vi "Global Chart List.vi"(7 "Action":T1=enum."Append to Charts", 10 "Value":dbl, 11 "Chart Ref":refnum<class "LQChart.lvclass">) -> ()   [LabVIEW 2014]
doc: "An Action Engine that registers and updates the global list of charts, which are created dynamically (at run-time) in this application.\n\n\nCopyright (c) 2019 Sze Howe Koh.\nThis code is licensed under the MIT license."
uses:
  Global Chart List Action.ctl
  <vilib>/addons/LQ/LQ Extras/LQChart/LQChart.lvclass
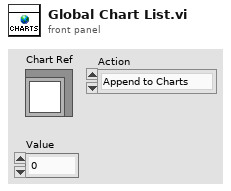
[diagram p1: front panel]
types:
  T1 = typedef "Global Chart List Action.ctl" = enum16{"Clear", "Register Chart", "Append to Charts"}
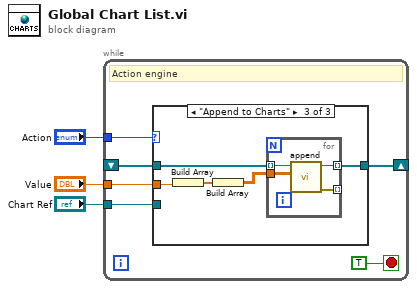
[diagram p0: block diagram]
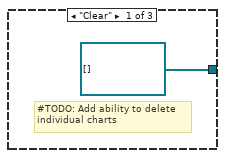
[diagram p2: hidden frame]
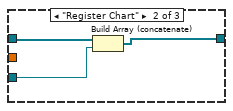
[diagram p3: hidden frame]
diagram:
  n1 = while {
    tunnel: "Action" -> [w8]
    shift-right: [w6] -> _
    shift-left: _ -> [w5]
    tunnel: "Chart Ref" -> [w7]
    tunnel: "Value" -> [w4]
    stop <- TRUE stop-if-true
    # "Action engine"
    n2 = case shown="\"Append to Charts\"" w8 {
      tunnel: w7 -> [_ w13 _]
      tunnel: [refnum<class "LQChart.lvclass">[] [] ("appended array") w11 w14] -> w6
      tunnel: w5 -> [_ w12 w18]
      tunnel: w4 -> [_ _ w17]
      frame "Clear" {
        # "#TODO: Add ability to delete\nindividual charts"
      }
      frame "Register Chart" {
        n3 = Build Array (concatenate)(w12, w13) -> (w11:refnum<class "LQChart.lvclass">[])
      }
      frame "Append to Charts" {
        n4 = Build Array(w17) -> (w16:dbl[])
        n5 = Build Array(w16) -> (w15:dbl[][])
        n6 = for {
          tunnel: w18 -> [w22] mode=indexing
          tunnel: w15 -> [w21]
          tunnel: [w20] -> _ mode=indexing
          tunnel: [w19] -> w14 mode=indexing
          n7 = call <vilib>:"append.vi"("values"=w21, "LQChart In"=w22) -> ("Error Out"=w20:errorcluster, "LQChart Out"=w19:refnum<class "LQChart.lvclass">)  [unwired: 8 in]
        }
      }
    }
  }
